vi "Handle Help.vi"(8 "error in (no error)":errorcluster, 10 "Command":variant, 11 "Instrument in":refnum<class "Instrument.lvclass">) -> (0 "error out":errorcluster, 2 "Help":variant, 3 "Instrument out":refnum<class "Instrument.lvclass">)   [LabVIEW 2019, in "Instrument.lvclass"]
uses:
  Instrument.lvclass
  Help/Help.lvclass
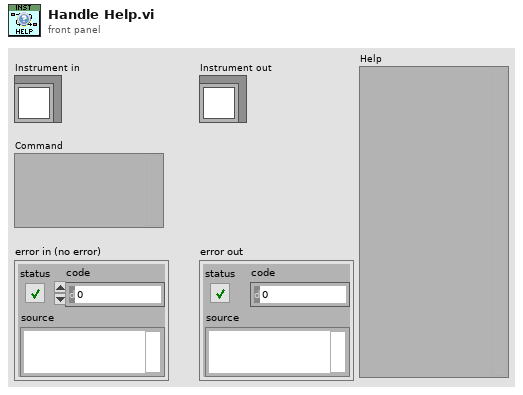
[diagram p1: front panel]
types:
  T1 = typedef "Help.lvclass/Help--cluster.ctl" = cluster{"command":string, "command description":string, "request cluster":variant, "response cluster":variant}
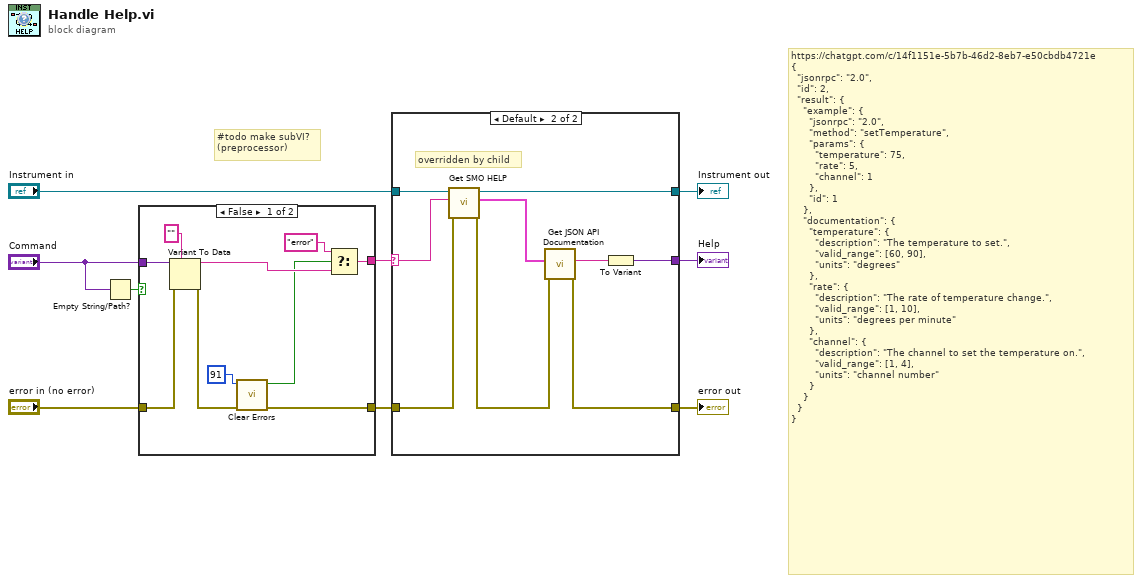
[diagram p0: block diagram]
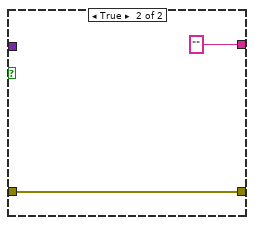
[diagram p2: hidden frame]
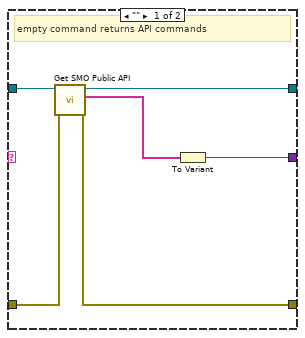
[diagram p3: hidden frame]
diagram:
  # "#todo make subVI?\n(preprocessor)"
  # "https://chatgpt.com/c/14f1151e-5b7b-46d2-8eb7-e50cbdb4721e\n{\n  \"jsonrpc\": \"2.0\",\n  \"id\": 2,\n  \"result\": {\n    \"example\": {\n      \"jsonrpc\": \"2.0\",\n      \"method\": \"setTemperature\",\n      \"params\": {\n        \"temperature\": 75,\n        \"rate\": 5,\n        \"channel\": 1\n      },\n      \"id\": 1\n    },\n    \"documentation\": {\n      \"temperature\": {\n        \"description\": \"The temperature to set.\",\n        \"valid_range\": [60, 90],\n        \"units\": \"degrees\"\n      },\n      \"rate\": {\n        \"description\": \"The rate of temperature change.\",\n        \"valid_range\": [1, 10],\n        \"units\": \"degrees per minute\"\n      },\n      \"channel\": {\n        \"description\": \"The channel to set the temperature on.\",\n        \"valid_range\": [1, 4],\n        \"units\": \"channel number\"\n      }\n    }\n  }\n}"
  n1 = Empty String/Path?(string/path="Command") -> (empty?=w8:bool)
  n2 = case shown="False" w8 {
    tunnel: "error in (no error)" -> [w19 w21]
    tunnel: [w13 ""] -> w4
    tunnel: [w15 w21] -> w5
    tunnel: "Command" -> [w17 _]
    frame False {
      n3 = Variant To Data(error in=w19, type="", Variant=w17) -> (data=w14:string, error out=w16:errorcluster)
      n4 = call <vilib>:"Clear Errors.vi"("error in (no error)"=w16, "specific error code to clear (0: all)"=91) -> ("error out"=w15:errorcluster, "specific error cleared?"=w10:bool)  [unwired: 4 in]
      n5 = Select(t="error", s=w10, f=w14) -> (s? t:f=w13:string)
    }
    frame True {
    }
  }
  n6 = case shown="Default" w4 {
    selector: w4 -> [_ w30]
    tunnel: w5 -> [w23 w32]
    tunnel: [w27 w35] -> w3
    tunnel: [w24 w28] -> w2
    tunnel: "Instrument in" -> [w26 w34]
    tunnel: [w22 w33] -> w1
    frame "" {
      # "empty command returns API commands"
      n7 = call-dynamic "Get SMO Public API.vi"("error in (no error)"=w23, "Instrument in"=w26) -> ("error out"=w24:errorcluster, "commands"=w25:string[], "Instrument out"=w22:refnum<class "Instrument.lvclass">)  [unwired: 7 in]
      n8 = To Variant(anything=w25) -> (Variant=w27:variant)
    }
    frame Default {
      # "overridden by child"
      n9 = call-dynamic "Get SMO HELP.vi"("error in (no error)"=w32, "Command"=w30, "Instrument in"=w34) -> ("error out"=w31:errorcluster, "help cluster"=w29:T1, "Instrument out"=w33:refnum<class "Instrument.lvclass">)  [unwired: 6 in]
      n10 = call "Get JSON API Documentation.vi"("error in (no error)"=w31, "Help cluster"=w29) -> ("error out"=w28:errorcluster, "<JSON> API doc"=w36:string)  [unwired: 7 in, 1 out]
      n11 = To Variant(anything=w36) -> (Variant=w35:variant)
    }
  }
  "Help" <- w3
  "Instrument out" <- w1
  "error out" <- w2
